vi "添加测试.vi"() -> (3 "12":dbl)   [LabVIEW 2010]
panel:
  in  "?":dbl format="%#_11g"
  in  "添加":bool
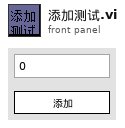
[diagram p1: front panel]
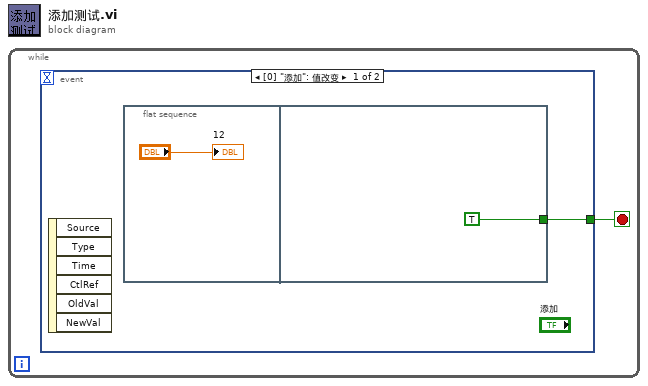
[diagram p0: block diagram]
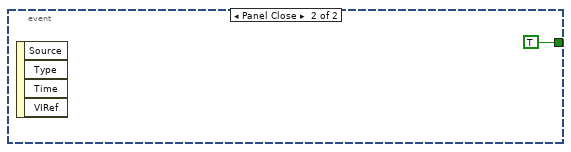
[diagram p2: hidden frame]
diagram:
  n1 = while {
    stop <- w1 stop-if-true
    n2 = event shown="[0] \"添加\": 值改变" {
      selector: _ -> [_ _]
      dyn-events: _ -> [_ _]
      timeout: _ -> [_ _]
      tunnel: [w2 TRUE] -> w1
      event "添加": Value Change {
        n3 = event-data() -> ()  [unwired: 1 in, 6 out]
        n4 = flat-sequence {
          tunnel: [TRUE ("添加")] -> w2
          frame #0 {
            "12" <- "?"
          }
          frame #1 {
          }
        }
      }
      event Panel Close {
        n5 = event-data() -> ()  [unwired: 1 in, 4 out]
      }
    }
  }
